vi "Configure Level.vi"(8 "Error In":errorcluster, 11 "Level":u8=7) -> (0 "Error Out":errorcluster)   [LabVIEW 2014, in "CF-Logger.lvlib"]
uses:
  CF-Logger.lvlib
  Private/_Logger Action.ctl
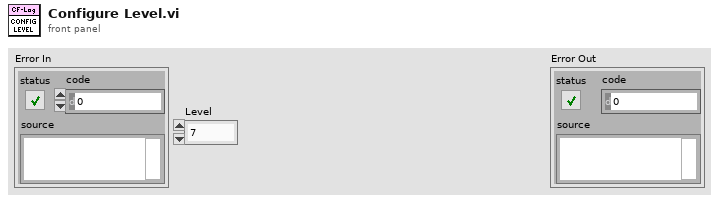
[diagram p1: front panel]
types:
  T1 = typedef "CF-Logger.lvlib/_Logger Action.ctl" = enum16{"Initialize", "Register", "Log", "Unregister", "Set Level", "Shutdown"}
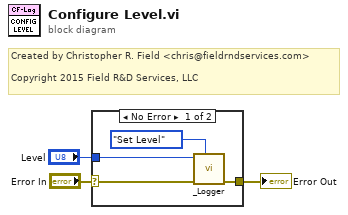
[diagram p0: block diagram]
diagram:
  # "Created by Christopher R. Field <chris@fieldrndservices.com>\n\nCopyright 2015 Field R&D Services, LLC"
  n1 = case shown="No Error" "Error In" {
    selector: "Error In" -> [w6 w8]
    tunnel: "Level" -> [w5 _]
    tunnel: [w4 w8] -> w1
    frame No Error {
      n2 = call "_Logger.vi"("Action"=_Logger_Action."Set Level", "Error In"=w6, "Value In"=w5) -> ("Error Out"=w4:errorcluster)  [unwired: 8 in]
    }
    frame Error {
    }
  }
  "Error Out" <- w1
